vi "Cron&EventTab@RedisStart__Parameter.vi"(1 "ParamterIn":string) -> (0 "ParamterOut":string)   [LabVIEW 2020]
panel:
  in  "RedisKey":string(combo)
  in  "Password":string(combo)
  in  "UserName":string(combo)
  in  "Port":string(combo)
  in  "Host":string(combo)
  in  "RedisTab":string(combo)
  in  "Confirm":bool
  # "RedisTab,RedisKey@Host:Port(,User:Password)"
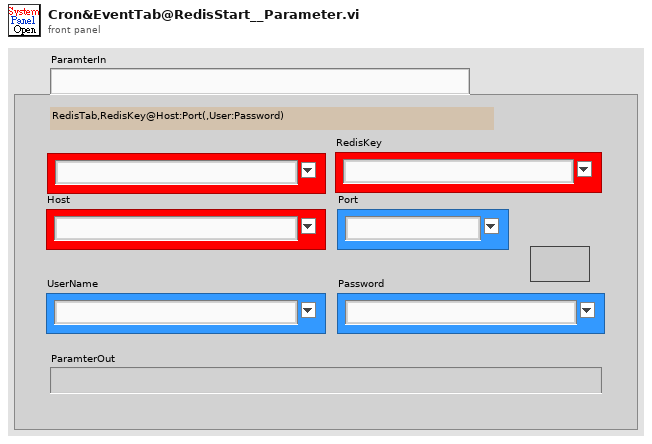
[diagram p1: front panel]
types:
  T1 = enum16{"Init", "Add", "Enable", "Disable", "Get", "UpdateVI"}
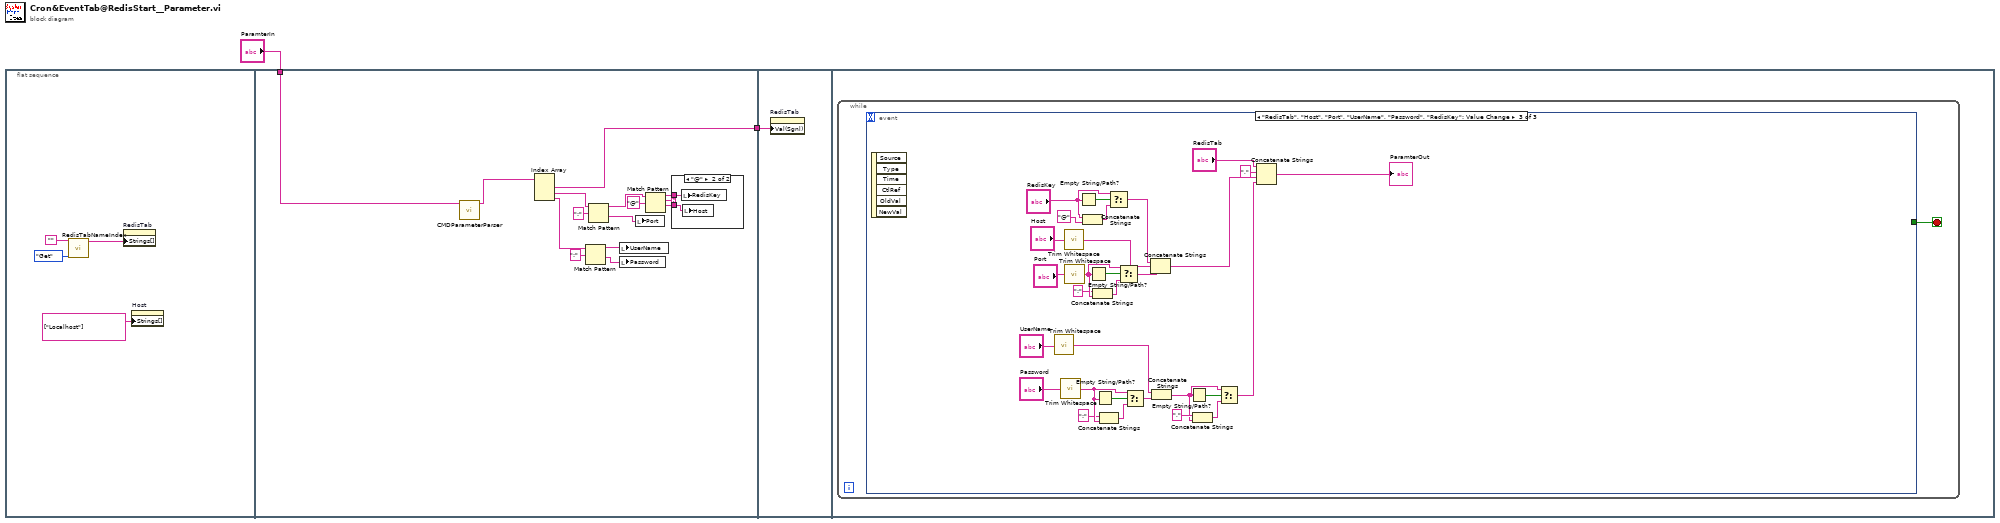
[diagram p0: block diagram]
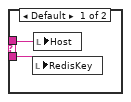
[diagram p2: hidden frame]
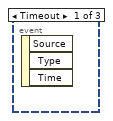
[diagram p3: hidden frame]
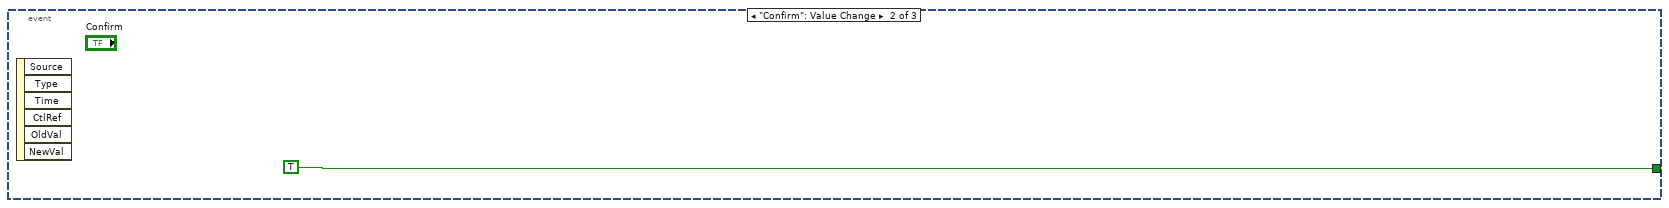
[diagram p4: hidden frame]
diagram:
  n1 = flat-sequence {
    tunnel: "ParamterIn" -> [w21]
    tunnel: [w19] -> w1
    tunnel: w1 -> [w26]
    frame #0 {
      n2 = call "RedisTabNameIndex.vi"("OP"=T1."Get", "RedisTabName"="") -> ("RedisTabNameS"=w3:string[])  [unwired: 5 in, 4 out]
      n3 = property on="RedisTab" class="CmbBox"("Strings[]"=w3) -> ()  [unwired: 2 in, 2 out]
      n4 = property on="Host" class="CmbBox"("Strings[]"=string[] ["Localhost"] ("Strings []")) -> ()  [unwired: 2 in, 2 out]
    }
    frame #1 {
      n5 = call "CMDParameterParser.vi"("CMDParameter"=w21) -> ("Input"=w20:string[])  [unwired: 8 in, 2 out]
      n6 = Index Array(array=w20) -> (element #1=w19:string, element #2=w18:string, element #3=w12:string)  [unwired: 3 in]
      n7 = Match Pattern(string=w12, regular expression=":") -> (before substring=w11:string, after substring=w10:string)  [unwired: 1 in, 2 out]
      n8 = Match Pattern(string=w18, regular expression=":") -> (before substring=w15:string, after substring=w14:string)  [unwired: 1 in, 2 out]
      n9 = local write "UserName"(w11) -> ()
      n10 = local write "Password"(w10) -> ()
      n11 = local write "Port"(w14) -> ()
      n12 = Match Pattern(string=w15, regular expression="@") -> (before substring=w8:string, match substring=w9:string, after substring=w7:string)  [unwired: 1 in, 1 out]
      n13 = case shown="\"@\"" w9 {
        tunnel: w8 -> [w23 w25]
        tunnel: w7 -> [w22 w24]
        frame Default {
          n14 = local write "RedisKey"(w22) -> ()
          n15 = local write "Host"(w23) -> ()
        }
        frame "@" {
          n16 = local write "RedisKey"(w25) -> ()
          n17 = local write "Host"(w24) -> ()
        }
      }
    }
    frame #2 {
      n18 = property on="RedisTab" class="CmbBox"("Val(Sgnl)"=w26) -> ()  [unwired: 2 in, 2 out]
    }
    frame #3 {
      n19 = while {
        stop <- w27 stop-if-true
        n20 = event shown="[2] \"RedisTab\", \"Host\", \"Port\", \"UserName\", \"Password\", \"RedisKey\": Value Change" {
          selector: _ -> [_ _ _]
          dyn-events: _ -> [_ _ _]
          timeout: _ -> [_ _ _]
          tunnel: [_ TRUE _] -> w27
          event Timeout {
            n21 = event-data() -> ()  [unwired: 1 in, 3 out]
          }
          event "Confirm": Value Change {
            n22 = event-data() -> ()  [unwired: 1 in, 6 out]
          }
          event "RedisTab", "Host", "Port", "UserName", "Password", "RedisKey": Value Change {
            n23 = event-data() -> ()  [unwired: 1 in, 6 out]
            n24 = call <vilib>:"Trim Whitespace.vi"("string"="UserName") -> ("trimmed string"=w40:string)  [unwired: 1 in]
            n25 = call <vilib>:"Trim Whitespace.vi"("string"="Password") -> ("trimmed string"=w45:string)  [unwired: 1 in]
            n26 = call <vilib>:"Trim Whitespace.vi"("string"="Host") -> ("trimmed string"=w42:string)  [unwired: 1 in]
            n27 = call <vilib>:"Trim Whitespace.vi"("string"="Port") -> ("trimmed string"=w49:string)  [unwired: 1 in]
            n28 = Empty String/Path?(string/path="RedisKey") -> (empty?=w32:bool)
            n29 = Concatenate Strings("RedisKey", "@" ("string")) -> (w33:string)
            n30 = Empty String/Path?(string/path=w49) -> (empty?=w51:bool)
            n31 = Concatenate Strings(":" ("string"), w49) -> (w50:string)
            n32 = Empty String/Path?(string/path=w45) -> (empty?=w46:bool)
            n33 = Concatenate Strings(":" ("string"), w45) -> (w47:string)
            n34 = Select(t="RedisKey", s=w32, f=w33) -> (s? t:f=w31:string)
            n35 = Select(t=w49, s=w51, f=w50) -> (s? t:f=w43:string)
            n36 = Select(t=w45, s=w46, f=w47) -> (s? t:f=w41:string)
            n37 = Concatenate Strings(w31, w42, w43) -> (w39:string)
            n38 = Concatenate Strings(w40, w41) -> (w36:string)
            n39 = Empty String/Path?(string/path=w36) -> (empty?=w38:bool)
            n40 = Concatenate Strings("," ("string"), w36) -> (w35:string)
            n41 = Select(t=w36, s=w38, f=w35) -> (s? t:f=w34:string)
            n42 = Concatenate Strings("RedisTab", "," ("string"), w39, w34) -> (→"ParamterOut":string)
          }
        }
      }
    }
  }
